vi "Read Saftey System Interlock.vi"(4 "error in":errorcluster) -> (0 "error out":errorcluster, 2 "Safety System Interlock":bool)   [LabVIEW 2015]
uses:
  <vilib>/DAQmx/read.llb/DAQmx Read (Digital Bool 1Line 1Point).vi
  <vilib>/DAQmx/write.llb/DAQmx Write (Digital Bool 1Line 1Point).vi
  <vilib>/DAQmx/miscellaneous.llb/DAQmx Fill In Error Info.vi
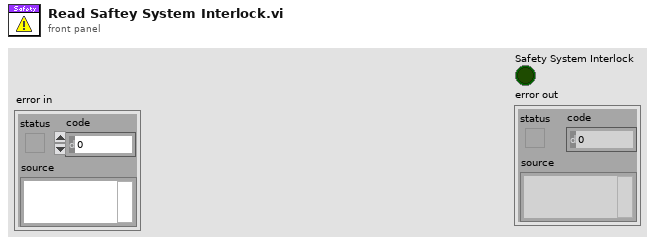
[diagram p1: front panel]
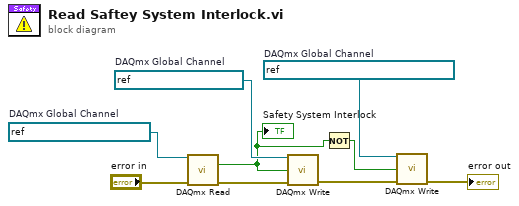
[diagram p0: block diagram]
diagram:
  w3 = refnum<k21> "DO12 System Reset Button LED"  # DAQmx Global Channel
  w8 = refnum<k21> "DO10 Interlock LED"  # DAQmx Global Channel
  w9 = refnum<k21> "DI1 Safety System trip"  # DAQmx Global Channel
  n1 = call-poly <vilib>:"DAQmx Read.vi"("task/channels in"=w9, "error in"="error in") -> ("data"=w2:bool, "error out"=w7:errorcluster)  [unwired: 11 in, 1 out]
  "Safety System Interlock" <- w2
  n2 = call-poly <vilib>:"DAQmx Write.vi"("task/channels in"=w8, "data"=w2, "error in"=w7) -> ("error out"=w5:errorcluster)  [unwired: 10 in, 2 out]
  n3 = Not(x=w2) -> (.not. x?=w1:bool)
  n4 = call-poly <vilib>:"DAQmx Write.vi"("task/channels in"=w3, "data"=w1, "error in"=w5) -> ("error out"=→"error out":errorcluster)  [unwired: 10 in, 2 out]
